vi "Test Lidar.vi"() -> ()   [LabVIEW 2017]
panel:
  out "XY Graph":cluster{dbl[], dbl[]}(graph)
  out "error out 2":errorcluster
  out "error out":errorcluster
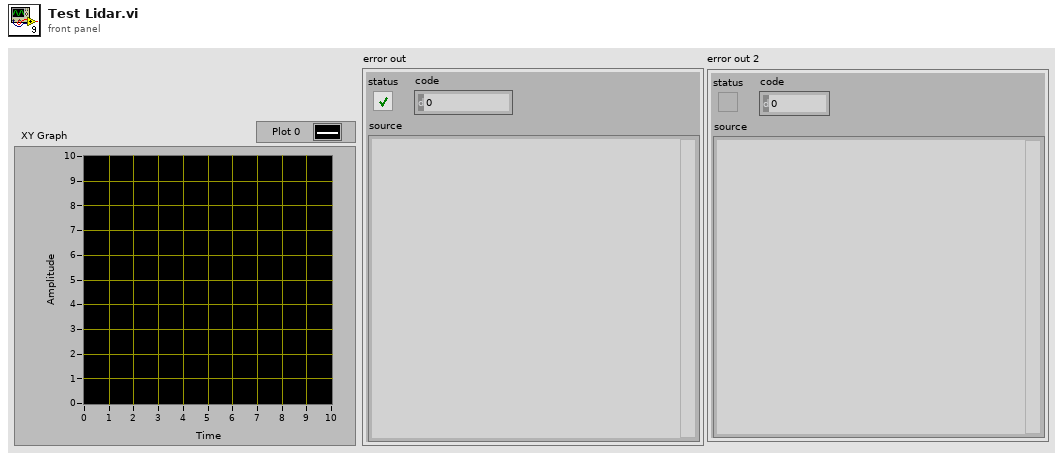
[diagram p1: front panel]
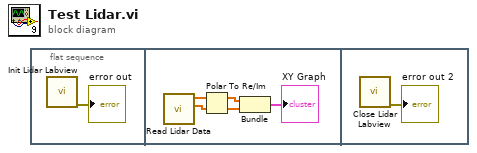
[diagram p0: block diagram]
diagram:
  n1 = flat-sequence {
    frame #0 {
      n2 = call "Init Lidar Labview.vi"() -> ("error out"=→"error out":errorcluster)  [unwired: 11 in]
    }
    frame #1 {
      n3 = call "Read Lidar Data.vi"() -> ("Direction"=w5:dbl[], "Magnitude"=w6:dbl[])  [unwired: 9 in, 1 out]
      n4 = Polar To Re/Im(2:w5, 3:w6) -> (0:w3:dbl[], 1:w4:dbl[])
      n5 = Bundle(w4, w3) -> (→"XY Graph":cluster{dbl[], dbl[]})  [unwired: 1 in]
    }
    frame #2 {
      n6 = call "Close Lidar Labview.vi"() -> ("error out"=→"error out 2":errorcluster)  [unwired: 11 in]
    }
  }
